vi "FFT_3_1_2.vi"() -> ()   [LabVIEW 2014]
uses:
  <vilib>/Analysis/2dsp.llb/Real FFT.vi
  <vilib>/measure/NI_MABase.lvlib
  <vilib>/Analysis/NI_AALPro.lvlib
panel:
  in  "Tab Control":T1(tab)
  in  "signal type":T2(ring)
  in  "reset signal":bool
  in  "offset":dbl format="%0.2p"
  in  "frequency":dbl=10.0 format="%0.2p"
  in  "amplitude":dbl=1.0 format="%0.2p"
  in  "phase":dbl format="%.2p"
  in  "square wave duty cycle (%)":dbl=50.0 format="%0.2f"
  in  "stop":bool
  in  "sampling info":cluster{"Fs":dbl, "#s":dbl}={"Fs"=1000.0, "#s"=1000.0} {"Fs" format="%.2p"}
  in  "offset 2":dbl format="%0.2p"
  in  "frequency 2":dbl=10.0 format="%0.2p"
  in  "amplitude 2":dbl=1.0 format="%0.2p"
  in  "phase 2":dbl format="%.2p"
  in  "square wave duty cycle (%) 2":dbl=50.0 format="%0.2f"
  in  "offset 3":dbl format="%0.2p"
  in  "frequency 3":dbl=10.0 format="%0.2p"
  in  "amplitude 3":dbl=1.0 format="%0.2p"
  in  "phase 3":dbl format="%.2p"
  in  "square wave duty cycle (%) 3":dbl=50.0 format="%0.2f"
  out "Waveform Graph":waveform(dbl)(graph)
  out "Waveform Graph 2":dbl[](graph)
  in  "shift?":bool
  out "error out":errorcluster
  out "error out 2":errorcluster
  out "error out 3":errorcluster
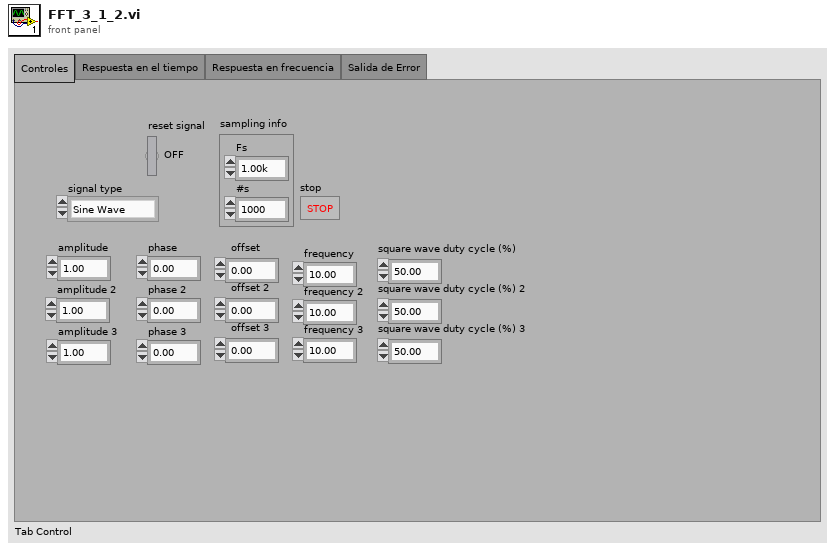
[diagram p1: front panel]
types:
  T1 = enum32{"Controles", "Respuesta en el tiempo", "Respuesta en frecuencia", "Salida de Error"}
  T2 = enum16{"Sine Wave", "Triangle Wave", "Square Wave", "Sawtooth Wave"}
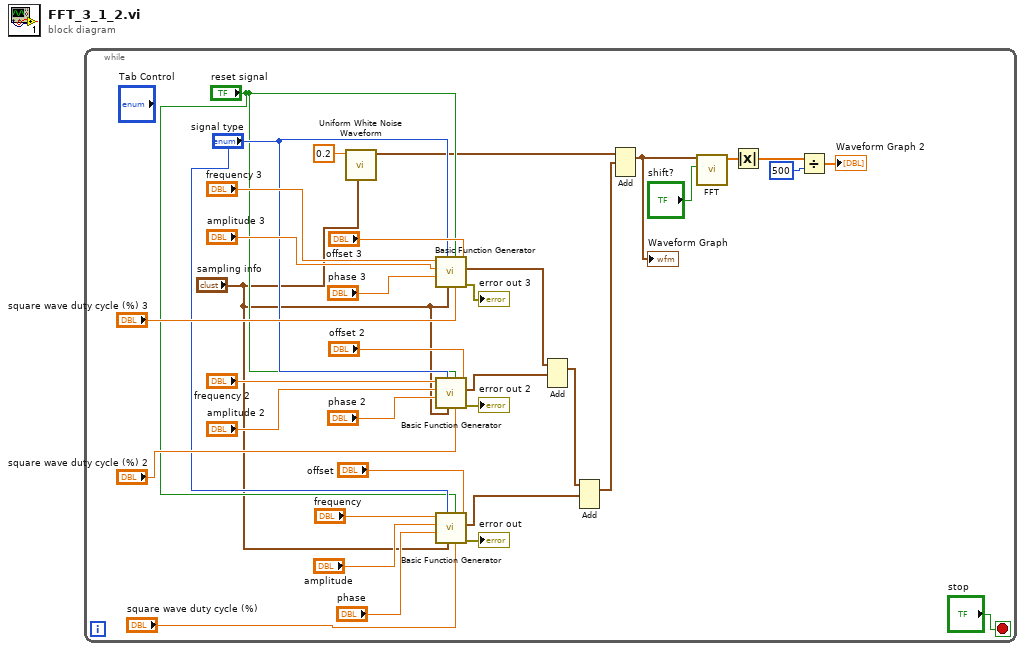
[diagram p0: block diagram]
diagram:
  n1 = while {
    stop <- "stop" stop-if-true
    n2 = call <vilib>:"Uniform White Noise Waveform.vi"("sampling info"="sampling info", "amplitude"=0.2) -> ("signal out"=w3:waveform(dbl))  [unwired: 8 in, 1 out]
    n3 = call <vilib>:"Basic Function Generator.vi"("offset"="offset 3", "square wave duty cycle (%)"="square wave duty cycle (%) 3", "reset signal"="reset signal", "sampling info"="sampling info", "signal type"="signal type", "phase"="phase 3", "amplitude"="amplitude 3", "frequency"="frequency 3") -> ("error out"=→"error out 3":errorcluster, "signal out"=w6:waveform(dbl))  [unwired: 1 in, 1 out]
    n4 = call <vilib>:"Basic Function Generator.vi"("offset"="offset 2", "square wave duty cycle (%)"="square wave duty cycle (%) 2", "reset signal"="reset signal", "sampling info"="sampling info", "signal type"="signal type", "phase"="phase 2", "amplitude"="amplitude 2", "frequency"="frequency 2") -> ("error out"=→"error out 2":errorcluster, "signal out"=w14:waveform(dbl))  [unwired: 1 in, 1 out]
    n5 = call <vilib>:"Basic Function Generator.vi"("offset"="offset", "square wave duty cycle (%)"="square wave duty cycle (%)", "reset signal"="reset signal", "sampling info"="sampling info", "signal type"="signal type", "phase"="phase", "amplitude"="amplitude", "frequency"="frequency") -> ("error out"=→"error out":errorcluster, "signal out"=w13:waveform(dbl))  [unwired: 1 in, 1 out]
    n6 = Add(1:w14, 2:w6) -> (0:w16:waveform(dbl))  [unwired: 1 in, 1 out]
    n7 = Add(1:w13, 2:w16) -> (0:w2:waveform(dbl))  [unwired: 1 in, 1 out]
    n8 = Add(1:w2, 2:w3) -> (0:w1:waveform(dbl))  [unwired: 1 in, 1 out]
    "Waveform Graph" <- w1
    n9 = call-poly <vilib>:"FFT.vi"("shift?"="shift?", "X"=w1) -> ("FFT {X}"=w12:cdb[])  [unwired: 8 in, 1 out]
    n10 = Absolute Value(x=w12) -> (abs(x)=w9:dbl[])
    n11 = Divide(x=w9, y=500) -> (x/y=→"Waveform Graph 2":dbl[])
  }
